vi "Alpha 4.1.vi"() -> ()   [LabVIEW 2011]
uses:
  <vilib>/vision/NI_Vision_Development_Module.lvlib
panel:
  in  "Color Plane":i32(ring)=1 items=["Red", "Green", "Blue", "Hue", "Saturation", "Luminance", "Value", "Intensity"]
  in  "Browse":bool
  in  "Stop":bool
  in  "Tab":enum32{"Parse", "Enhance Image", "Threshold"}(tab)
  out "Path":path
  out "Image":T1(plugin-control)
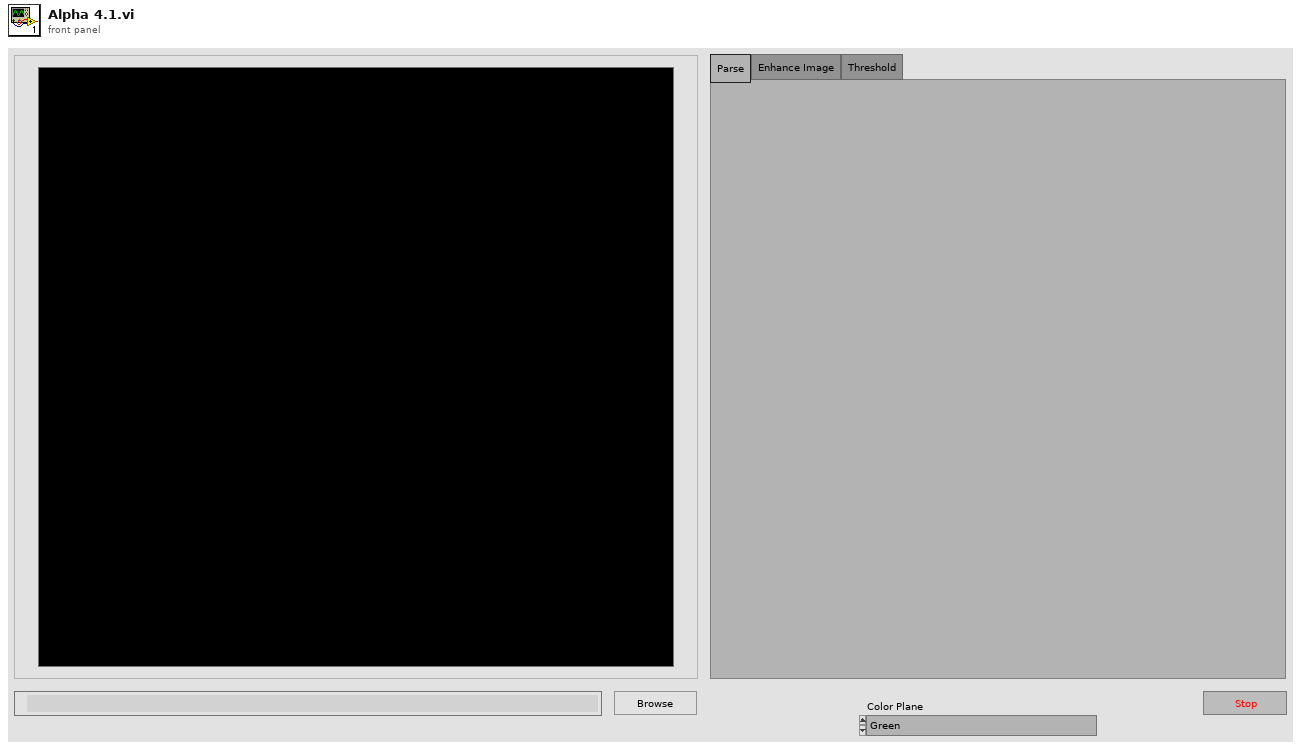
[diagram p1: front panel]
types:
  T1 = typedef "IMAQ Image.ctl" = refnum<image>
  T2 = typedef "Image Type" = u32
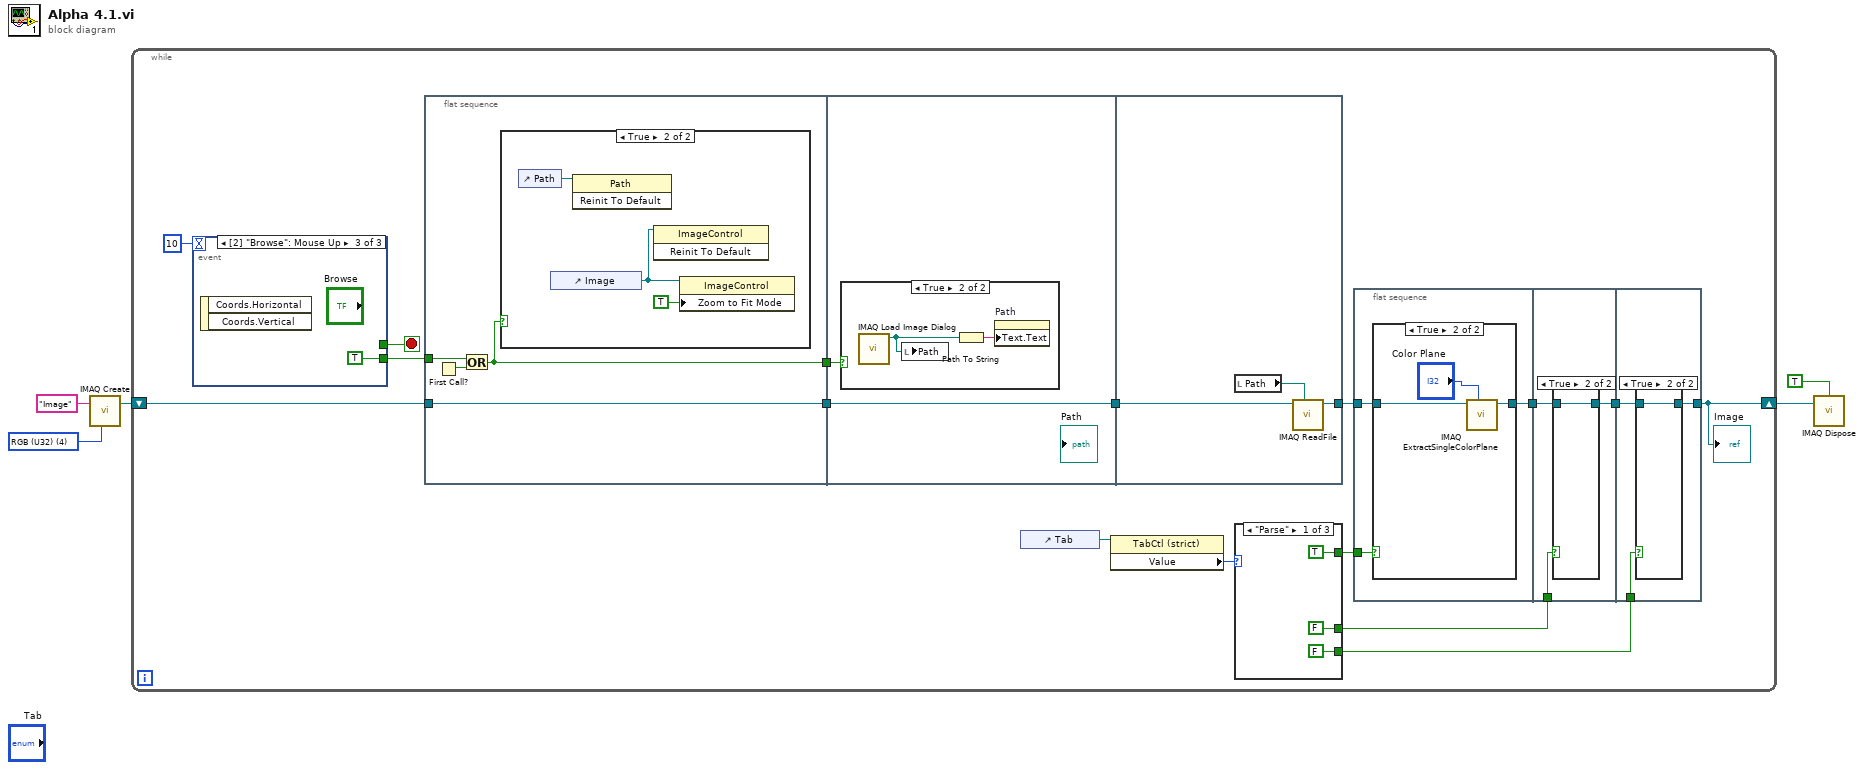
[diagram p0: block diagram]
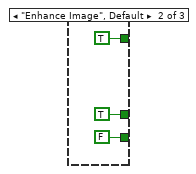
[diagram p5: hidden frame]
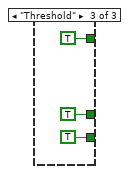
[diagram p6: hidden frame]
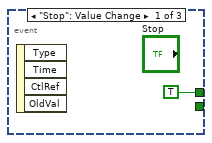
[diagram p9: hidden frame]
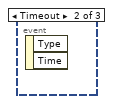
[diagram p10: hidden frame]
diagram:
  w4 = T2 4 items=["Grayscale (U8)", "Grayscale (I16)", "Grayscale (SGL)", "Complex (CSG)", "RGB (U32)", "HSL (U32)", "RGB (U64)", "Grayscale (U16)"] ("Image Type")
  n1 = call "IMAQ Create"("Image Name"="Image", "Image Type"=w4) -> ("New Image"=w3:T1)  [unwired: 3 in, 1 out]
  n2 = while {
    shift-right: [w8] -> w2
    shift-left: w3 -> [w20]
    stop <- w21 stop-if-true
    n3 = event shown="[2] \"Browse\": Mouse Up" {
      selector: _ -> [_ _ _]
      dyn-events: _ -> [_ _ _]
      timeout: 10 -> [_ _ _]
      tunnel: [TRUE _ _] -> w21
      tunnel: [_ _ TRUE] -> w17
      event "Stop": Value Change {
        n4 = event-data() -> ()  [unwired: 1 in, 4 out]
      }
      event Timeout {
        n5 = event-data() -> ()  [unwired: 1 in, 2 out]
      }
      event "Browse": Mouse Up {
        n6 = event-data() -> ()  [unwired: 1 in, 2 out]
      }
    }
    n7 = flat-sequence {
      tunnel: w20 -> [w51]
      tunnel: [w51] -> w19
      tunnel: w17 -> [w50]
      tunnel: [w48] -> w16
      tunnel: w19 -> [w56]
      tunnel: [w56] -> w18
      tunnel: w16 -> [w55]
      tunnel: w18 -> [w61]
      tunnel: [w60] -> w10
      frame #0 {
        n8 = First Call?() -> (First Call?: T/F=w49:bool)
        n9 = Or(x=w50, y=w49) -> (x .or. y?=w48:bool)
        n10 = case shown="True" w48 {
          frame False {
          }
          frame True {
            n11 = control-ref of="Path"() -> (w54:refnum<vi>)
            n12 = control-ref of="Image"() -> (w52:refnum<vi>)
            n13 = invoke class="Path" method="Reinit To Default"(reference=w54) -> ()  [unwired: 2 in, 3 out]
            n14 = invoke class="ImageControl" method="Reinit To Default"(reference=w52) -> ()  [unwired: 2 in, 3 out]
            n15 = property class="ImageControl"(reference=w52, "Zoom to Fit Mode"=TRUE) -> ()  [unwired: 1 in, 2 out]
          }
        }
      }
      frame #1 {
        n16 = case shown="True" w55 {
          frame False {
          }
          frame True {
            n17 = call "IMAQ Load Image Dialog"() -> ("Path"=w57:path)  [unwired: 9 in, 2 out]
            n18 = local write "Path"(w57) -> ()
            n19 = Path To String(path=w57) -> (string=w58:string)
            n20 = property on="Path" class="Path"("Text.Text"=w58) -> ()  [unwired: 2 in, 2 out]
          }
        }
      }
      frame #2 {
        n21 = local read "Path"() -> (w59:path)
        n22 = call "IMAQ ReadFile"("File Path"=w59, "Image"=w61) -> ("Image Out"=w60:T1)  [unwired: 5 in, 4 out]
      }
    }
    n23 = control-ref of="Tab"() -> (w14:refnum<vi>)
    n24 = property class="TabCtl (strict)"(reference=w14) -> ("Value"=w13:enum32{"Parse", "Enhance Image", "Threshold"})  [unwired: 1 in, 2 out]
    n25 = case shown="\"Parse\"" w13 {
      tunnel: [TRUE TRUE TRUE] -> w12
      tunnel: [FALSE TRUE TRUE] -> w11
      tunnel: [FALSE FALSE TRUE] -> w6
      frame "Parse" {
      }
      frame "Enhance Image", Default {
      }
      frame "Threshold" {
      }
    }
    n26 = flat-sequence {
      tunnel: w12 -> [w24]
      tunnel: w10 -> [w23]
      tunnel: [w22] -> w9
      tunnel: w11 -> [w31]
      tunnel: w9 -> [w30]
      tunnel: [w29] -> w7
      tunnel: [w36] -> w8
      tunnel: w7 -> [w35]
      tunnel: w6 -> [w34]
      frame #0 {
        n27 = case shown="True" w24 {
          tunnel: w23 -> [w25 w28]
          tunnel: [w25 w27] -> w22
          frame False {
          }
          frame True {
            n28 = call "IMAQ ExtractSingleColorPlane"("Color Plane"="Color Plane", "Image Src"=w28) -> ("Image Dst Out"=w27:T1)  [unwired: 8 in, 1 out]
          }
        }
      }
      frame #1 {
        n29 = case shown="True" w31 {
          tunnel: w30 -> [w32 w33]
          tunnel: [w32 w33] -> w29
          frame False {
          }
          frame True {
          }
        }
      }
      frame #2 {
        n30 = case shown="True" w34 {
          tunnel: w35 -> [w37 w38]
          tunnel: [w37 w38] -> w36
          frame False {
          }
          frame True {
          }
        }
      }
    }
    "Image" <- w8
  }
  n31 = call "IMAQ Dispose"("All Images? (No)"=TRUE, "Image"=w2) -> ()  [unwired: 4 in, 1 out]
